vi "STATUS.vi"(8 "error in (no error)":errorcluster, 11 "refnum in":T2) -> (0 "error out":errorcluster, 1 "Status":T1, 2 "data out":string, 3 "refnum out":T2, 4 "question out":string)   [LabVIEW 2021, in "Korad KA3305P.lvlib"]
uses:
  Korad KA3305P.lvlib
  Reference.ctl
  Status.ctl
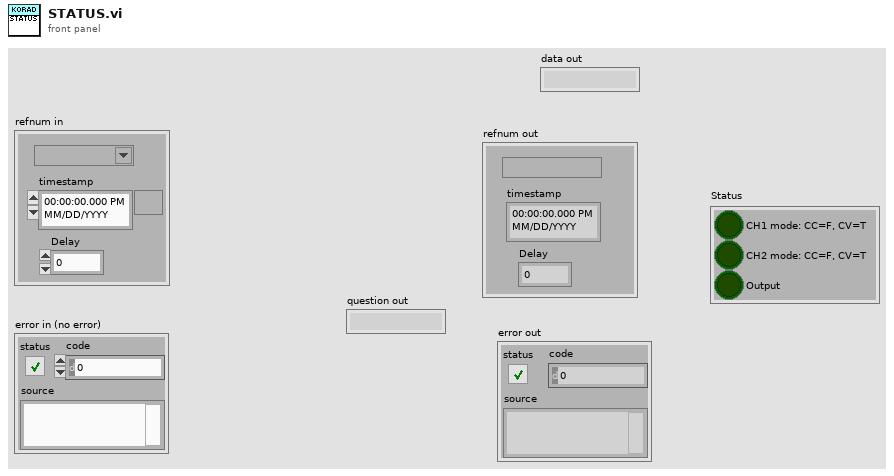
[diagram p1: front panel]
types:
  T1 = typedef "Korad KA3305P.lvlib/Status.ctl" = cluster{"CH1 mode: CC=F, CV=T":bool, "CH2 mode: CC=F, CV=T":bool, "Output":bool}
  T2 = typedef "Korad KA3305P.lvlib/Reference.ctl" = cluster{"refnum":refnum<visa-resource-name>, "timestamp":timestamp, "Delay":dbl}
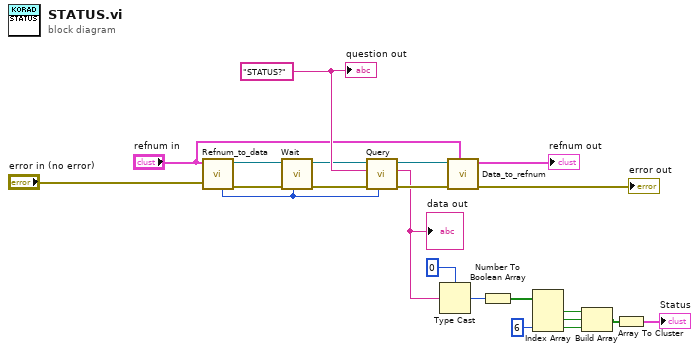
[diagram p0: block diagram]
diagram:
  w19 = "STATUS?" ("string")
  n1 = call "Refnum_to_data.vi"("error in (no error)"="error in (no error)", "refnum in"="refnum in") -> ("error out"=w12:errorcluster, "DAQ refnum out"=w13:refnum<visa-resource-name>, "delay out"=w22:u32)  [unwired: 7 in]
  n2 = call "Wait.vi"("milliseconds to wait"=w22, "error in (no error)"=w12, "refnum in"=w13) -> ("error out"=w18:errorcluster, "refnum out"=w17:refnum<visa-resource-name>)  [unwired: 7 in]
  n3 = call "Query.vi"("delay (55ms)"=w22, "error in (no error)"=w18, "data in"=w19, "refnum in"=w17) -> ("error out"=w21:errorcluster, "data out"=w10:string, "refnum out"=w20:refnum<visa-resource-name>)  [unwired: 5 in]
  "data out" <- w10
  n4 = Type Cast(type=u8 0, x=w10) -> (*(type *) &x=w8:u8)
  n5 = call "Data_to_refnum.vi"("refnum in"="refnum in", "error in (no error)"=w21, "DAQ refnum in"=w20) -> ("error out"=→"error out":errorcluster, "refnum out"=→"refnum out":T2)  [unwired: 7 in]
  n6 = Number To Boolean Array(number=w8) -> (Boolean array=w7:bool[])
  n7 = Index Array(array=w7, index #3=6 ("index")) -> (element #1=w5:bool, element #2=w4:bool, element #3=w3:bool)  [unwired: 2 in]
  n8 = Build Array(w5, w4, w3) -> (w2:bool[])
  n9 = Array To Cluster(array=w2) -> (cluster=→"Status":cluster{"[0]":bool, "[1]":bool, "[2]":bool})
  "question out" <- w19
